vi "Monitoring Keyboard and Mouse Activity.vi"() -> ()   [LabVIEW 2023]
doc: "This VI shows how to use the Input Device Control VIs. It displays keyboard and mouse activity while the VI is running. The Input Device Control VIs can also be used to display joystick information."
uses:
  <vilib>/Utility/inputDevices.llb/keyboardAcquire.vi
  <vilib>/Utility/inputDevices.llb/mouseAcquire.vi
  <vilib>/Utility/inputDevices.llb/closeKeyboard.vi
  <vilib>/Utility/inputDevices.llb/closeMouse.vi
panel:
  out "Keys Pressed":T1(array[ring])
  out "Vertical Mouse Position":i32
  out "Horizontal Mouse Position":i32
  out "Mouse Button 2":bool
  out "Mouse Button 1":bool
  in  "Stop":bool
  # "Overview: Demonstrates the use of the Input Device Control VIs to monitor mouse and keyboard actions.\nRequirements: Windows or Linux\nInstructions:\n1. Run the VI.\n2. Observe the values of the indicators update as you press keyboard keys, change the mouse position, and click mouse buttons.\n3. Click Stop to stop the VI."
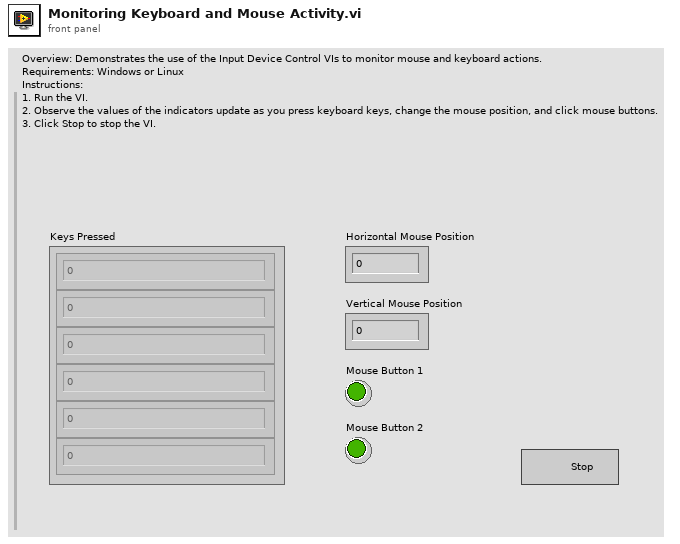
[diagram p1: front panel]
types:
  T1 = enum16{"0", "1", "2", "3", "4", "5", "6", "7", "8", "9", "A", "B", "C", "D", "E", "F", "G", "H", "I", "J", "K", "L", "M", "N", "O", "P", "Q", "R", "S", "T", "U", "V", "W", "X", "Y", "Z", "F1", "F2", "F3", "F4", "F5", "F6", "F7", "F8", "F9", "F10", "F11", "F12", "F13", "F14", "F15", "ADD", "BACK", "BACKSLASH", "CAPITAL", "COMMA", "DECIMAL", "DELETE", "DIVIDE", "DOWN", "END", "EQUALS", "ESCAPE", "GRAVE (`)", "HOME", "INSERT", "LBRACKET", "LCONTROL", "LEFT", "L ALT", "LSHIFT", "LWIN", "MINUS", "MULTIPLY", "NEXT", "NUMLOCK", "NUMPAD_0", "NUMPAD_1", "NUMPAD_2", "NUMPAD_3", "NUMPAD_4", "NUMPAD_5", "NUMPAD_6", "NUMPAD_7", "NUMPAD_8", "NUMPAD_9", "PAUSE", "PERIOD", "PRIOR (PG UP)", "RBRACKET", "RCONTROL", "RETURN", "RIGHT", "R ALT", "RSHIFT", "RWIN", "SCROLL", "SEMICOLON", "SLASH", "SPACE", "SUBTRACT", "TAB", "UP", "ENTER (num pad)", "' (quote)"}[]
  T2 = cluster{"Horizontal":i32, "Vertical":i32, "Scrolling":i32}
  T3 = cluster{"button 1":bool, "button 2":bool, "button 3":bool, "button 4":bool}
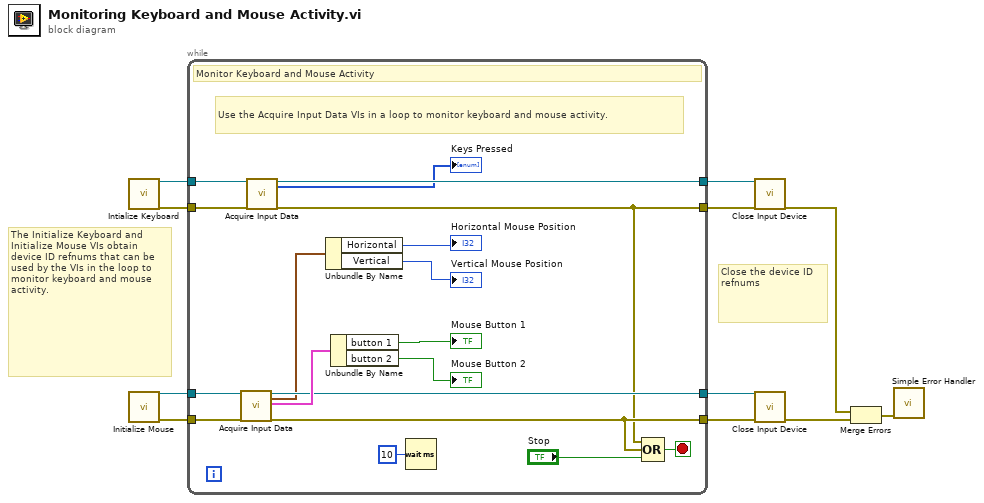
[diagram p0: block diagram]
diagram:
  # "Close the device ID refnums"
  # "The Initialize Keyboard and Initialize Mouse VIs obtain device ID refnums that can be used by the VIs in the loop to monitor keyboard and mouse activity."
  n1 = call <vilib>:"Intialize Keyboard.vi"() -> ("error out"=w9:errorcluster, "device ID"=w11:refnum<k1>)  [unwired: 1 in, 9 out]
  n2 = call <vilib>:"Initialize Mouse.vi"() -> ("error out"=w8:errorcluster, "device ID"=w10:refnum<k1>)  [unwired: 1 in, 9 out]
  n3 = while {
    tunnel: [w13] -> w3
    tunnel: [w23] -> w4
    tunnel: [w12] -> w5
    tunnel: w8 -> [w27]
    tunnel: w9 -> [w28]
    tunnel: w10 -> [w29]
    tunnel: [w24] -> w6
    tunnel: w11 -> [w22]
    stop <- w14 stop-if-true
    # "Use the Acquire Input Data VIs in a loop to monitor keyboard and mouse activity."
    # "Monitor Keyboard and Mouse Activity"
    n4 = call-poly <vilib>:"Acquire Input Data.vi"("device ID"=w29, "error in (no error)"=w27) -> ("device ID"=w23:refnum<k1>, "axis info"=w19:T2, "button info"=w26:T3, "error out"=w13:errorcluster)  [unwired: 1 in, 13 out]
    n5 = call-poly <vilib>:"Acquire Input Data.vi"("device ID"=w22, "error in (no error)"=w28) -> ("device ID"=w24:refnum<k1>, "keys pressed"=→"Keys Pressed":T1, "error out"=w12:errorcluster)  [unwired: 15 out]
    n6 = Unbundle By Name(w19) -> ("Horizontal"=→"Horizontal Mouse Position":i32, "Vertical"=→"Vertical Mouse Position":i32)
    n7 = Unbundle By Name(w26) -> ("button 1"=→"Mouse Button 1":bool, "button 2"=→"Mouse Button 2":bool)
    n8 = Wait (ms)(milliseconds to wait=u32 10) -> ()  [unwired: 1 out]
    n9 = Compound Arithmetic op=OR(w12, w13, "Stop") -> (w14:bool)
  }
  n10 = call-poly <vilib>:"Close Input Device.vi"("error in (no error)"=w5, "device ID"=w6) -> ("error out"=w1:errorcluster)  [unwired: 8 out]
  n11 = call-poly <vilib>:"Close Input Device.vi"("error in (no error)"=w3, "device ID"=w4) -> ("error out"=w2:errorcluster)  [unwired: 8 out]
  n12 = Merge Errors(w1, w2) -> (w7:errorcluster)
  n13 = call <vilib>:"Simple Error Handler.vi"("error in (no error)"=w7) -> ()  [unwired: 4 in, 5 out]
